vi "Name Value Remove Group Zero Case.vi"(0 "Tags Array":string[][][](array[string]), 7 "Boolean Refs Array":refnum<vi>[](array[refnum])) -> (4 "Updated Tag Array":string[][][](array[string]), 15 "Current Tags":string[][](array[string]))   [LabVIEW 2020]
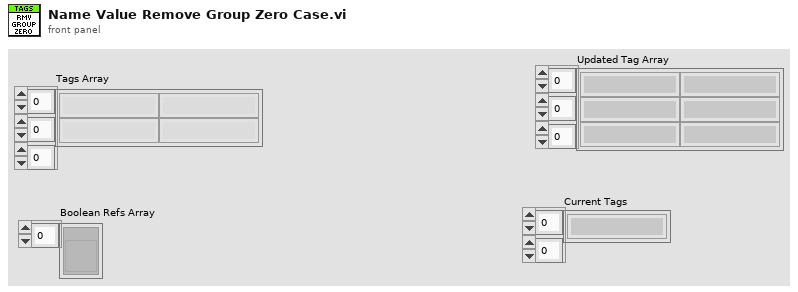
[diagram p1: front panel]
types:
  T1 = enum8{"Enabled", "Disabled", "Disabled and Grayed Out"}
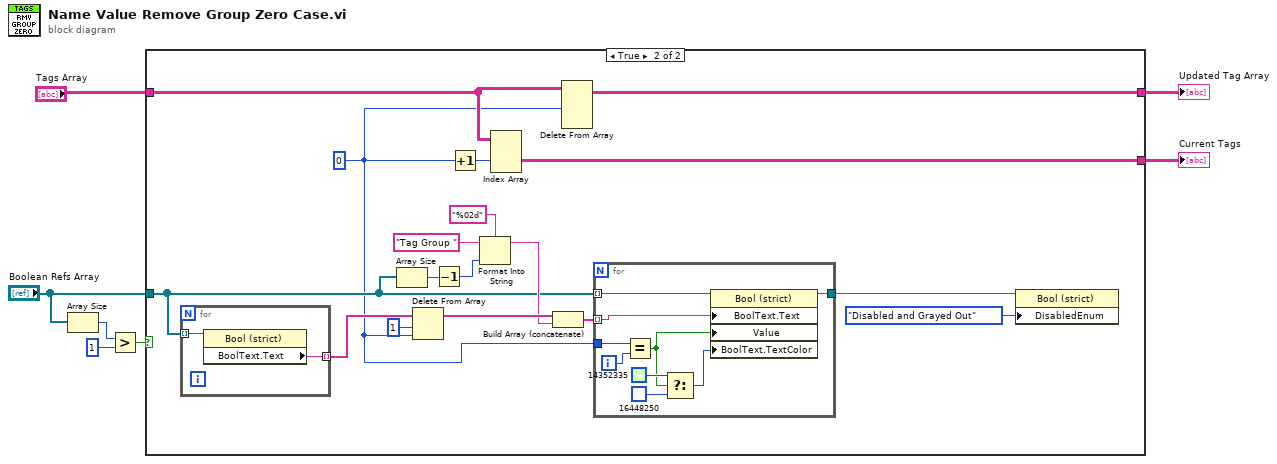
[diagram p0: block diagram]
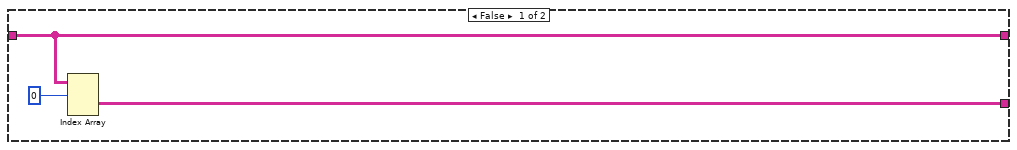
[diagram p2: hidden frame]
diagram:
  n1 = Array Size(array="Boolean Refs Array") -> (size(s)=w6:i32)
  n2 = Greater?(x=w6, y=1) -> (0:w4:bool)
  n3 = case shown="True" w4 {
    tunnel: "Boolean Refs Array" -> [_ w16]
    tunnel: "Tags Array" -> [w10 w14]
    tunnel: [w10 w13] -> w2
    tunnel: [w9 w11] -> w1
    frame False {
      n4 = Index Array(array=w10, index (dim 0)=0 ("disabled index (col)")) -> (element=w9:string[][])  [unwired: 2 in]
    }
    frame True {
      w12 = 0 ("Group Index")
      n5 = for {
        tunnel: w16 -> [w29] mode=indexing
        tunnel: [w28] -> w15 mode=indexing
        n6 = property class="Bool (strict)"(reference=w29) -> ("BoolText.Text"=w28:string)  [unwired: 1 in, 2 out]
      }
      n7 = Array Size(array=w16) -> (size(s)=w23:i32)
      n8 = Delete From Array(array=w15, length=1, index=w12) -> (array with subset deleted=w26:string[])  [unwired: 1 out]
      n9 = Decrement(x=w23) -> (x-1=w20:i32)
      n10 = Increment(x=w12) -> (x+1=w17:i32)
      n11 = Format Into String(format string="%02d", initial string="Tag Group ", w20) -> (resulting string=w22:string)  [unwired: 1 in, 1 out]
      n12 = Index Array(array=w14, index (dim 1)=w17) -> (element=w11:string[][])  [unwired: 2 in]
      n13 = Build Array (concatenate)(w26, w22) -> (w21:string[])
      n14 = Delete From Array(array=w14, index (dim 0)=w12) -> (array with subset deleted=w13:string[][][])  [unwired: 3 in, 1 out]
      n15 = for {
        tunnel: w16 -> [w38] mode=indexing
        tunnel: w21 -> [w35] mode=indexing
        tunnel: w12 -> [w37]
        tunnel: [w30] -> w18
        i -> [w36]
        n16 = Equal?(x=w37, y=w36) -> (x = y?=w32:bool)
        n17 = Select(t=u32 14352335 ("Color Box"), s=w32, f=u32 16448250) -> (s? t:f=w31:u32)
        n18 = property class="Bool (strict)"(reference=w38, "BoolText.Text"=w35, "Value"=w32, "BoolText.TextColor"=w31) -> (reference out=w30:refnum<vi>)  [unwired: 1 in, 1 out]
      }
      n19 = property class="Bool (strict)"(reference=w18, "DisabledEnum"=T1."Disabled and Grayed Out" ("Disabled")) -> ()  [unwired: 1 in, 2 out]
    }
  }
  "Updated Tag Array" <- w2
  "Current Tags" <- w1
